vi "Parse Paths and Directories for Classes.vi"(7 "base path":path, 8 "error in (no error)":errorcluster, 11 "Array of paths (folders to scan or explicit files)":path[](array[path])) -> (0 "error out":errorcluster, 3 "All Files in Dir":path[](array[path]))   [LabVIEW 2015, in "Controller Actor.lvlib" / "Controller.lvclass"]
uses:
  Controller.lvclass
  <userlib>/_OpenG.lib/file/file.llb/File Exists - Scalar__ogtk.vi
  <userlib>/_OpenG.lib/file/file.llb/Strip Path Extension - Path__ogtk.vi
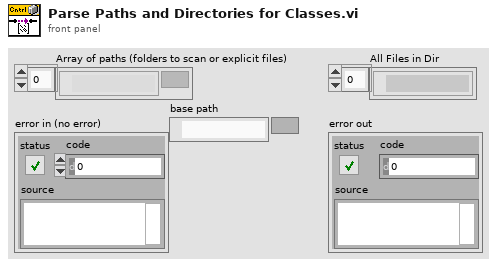
[diagram p1: front panel]
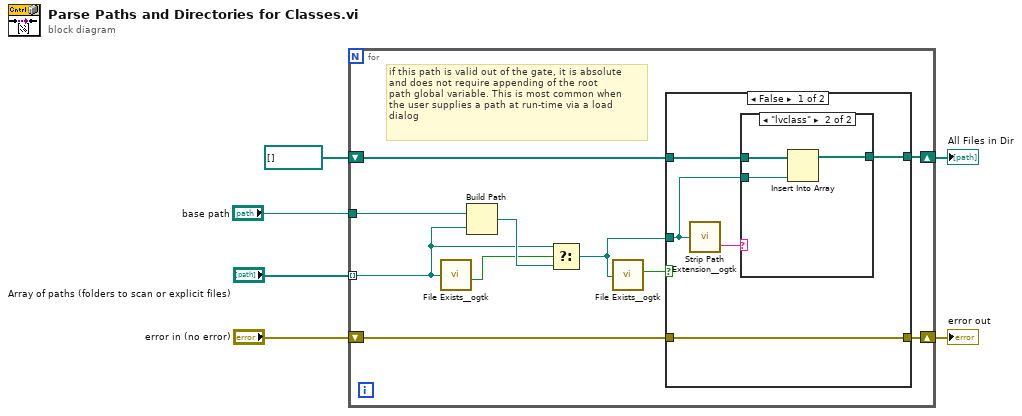
[diagram p0: block diagram]
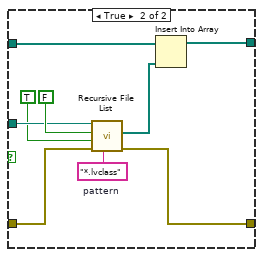
[diagram p3: hidden frame]
diagram:
  n1 = for {
    tunnel: "Array of paths (folders to scan or explicit files)" -> [w9] mode=indexing
    shift-right: [w14] -> w6
    shift-left: path[] [] ("All Files in Dir") -> [w15]
    shift-right: [w12] -> w5
    shift-left: "error in (no error)" -> [w13]
    tunnel: "base path" -> [w7]
    # "if this path is valid out of the gate, it is absolute\nand does not require appending of the root \npath global variable. This is most common when\nthe user supplies a path at run-time via a load\ndialog"
    n2 = call-poly <userlib>:"File Exists__ogtk.vi"("file path"=w9) -> ("exists"=w8:bool)  [unwired: 6 in, 1 out]
    n3 = Build Path(base path=w7, name or relative path=w9) -> (appended path=w11:path)
    n4 = Select(t=w9, s=w8, f=w11) -> (s? t:f=w10:path)
    n5 = call-poly <userlib>:"File Exists__ogtk.vi"("file path"=w10) -> ("is directory"=w16:bool)  [unwired: 6 in, 1 out]
    n6 = case shown="False" w16 {
      tunnel: w10 -> [w17 w32]
      tunnel: w15 -> [w21 w30]
      tunnel: [w20 w29] -> w14
      tunnel: w13 -> [w19 w27]
      tunnel: [w19 w26] -> w12
      frame False {
        n7 = call-poly <userlib>:"Strip Path Extension__ogtk.vi"("path"=w17) -> ("extension"=w18:string)  [unwired: 1 out]
        n8 = case shown="\"lvclass\"" w18 {
          tunnel: w21 -> [w22 w25]
          tunnel: [w22 w24] -> w20
          tunnel: w17 -> [_ w23]
          frame Default {
          }
          frame "lvclass" {
            n9 = Insert Into Array "Insert Into Array"(array=w25, new element=w23) -> (w24:path[])  [unwired: 1 in]
          }
        }
      }
      frame True {
        w33 = "*.lvclass"  # pattern
        n10 = call <vilib>:"Recursive File List.vi"("pattern"=w33, "error in (no error)"=w27, "Continue Recursing on Error? (F)"=TRUE, "Treat LLBs as Folders?"=FALSE, "Folder Path"=w32) -> ("error out"=w26:errorcluster, "All Files in Dir"=w28:path[])  [unwired: 2 in, 3 out]
        n11 = Insert Into Array "Insert Into Array"(array=w30, new element=w28) -> (w29:path[])  [unwired: 1 in]
      }
    }
  }
  "All Files in Dir" <- w6
  "error out" <- w5
